vi "Histogram Main.vi"() -> ()   [LabVIEW 2022 SP3]
uses:
  Consumer Message.ctl
  <vilib>/Utility/file.llb/Write Delimited Spreadsheet (DBL).vi
  <vilib>/ErrorRing/Error Ring.xnode
panel:
  out "Histogram":cluster{"histogram":dbl[], "x axis":dbl[]}(graph)
  in  "bins":i32=20
  in  "signal":u16(ring) items=["uniform white", "uniform+uniform", "Gaussian white", "sine", "square"]
  out "Consumer Shutdown?":bool
  out "Backlog":u8(slide) scale=0.0..100.0
  in  "Snapshot":bool
  in  "Stop":bool
  # "Number of enqueued messages waiting to be processed"
  # "Current data being processed in consumer loop"
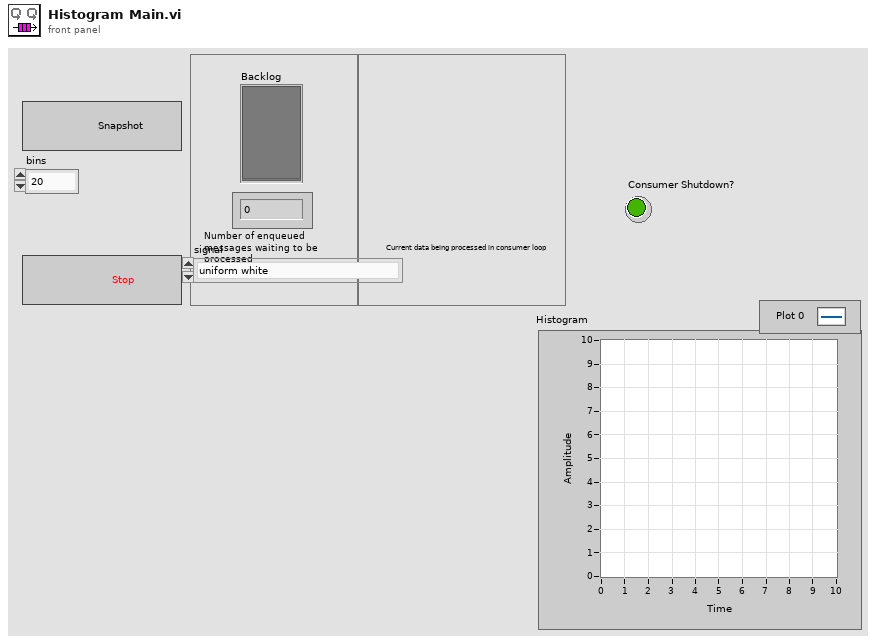
[diagram p1: front panel]
types:
  T1 = typedef "Consumer Message.ctl" = cluster{"Consumer State":string, "Boolean Data":bool, "Numeric Data":i32, "Signal":dbl[], "Error":errorcluster}
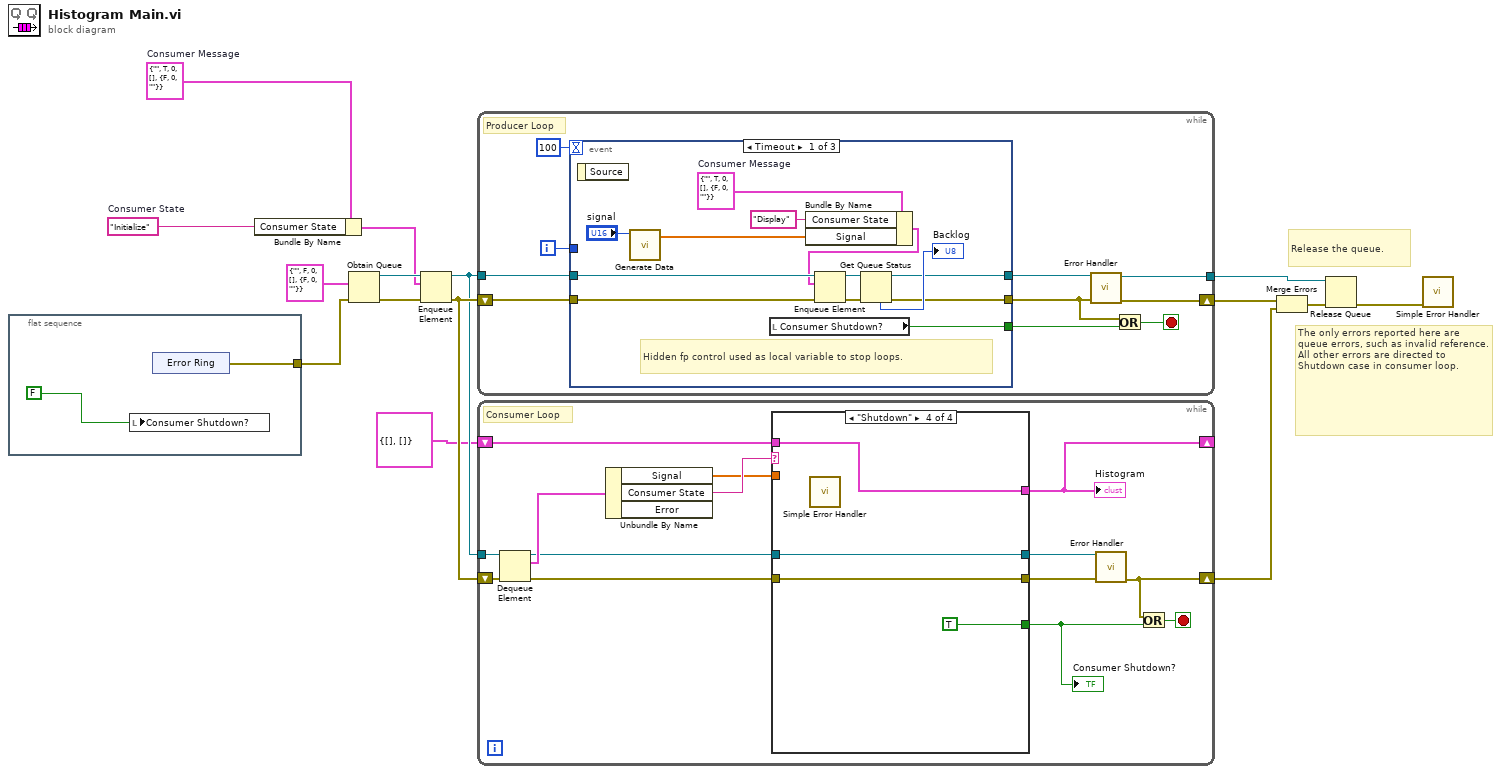
[diagram p0: block diagram]
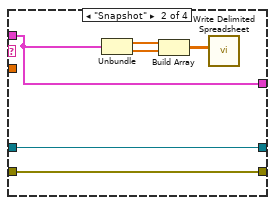
[diagram p3: hidden frame]
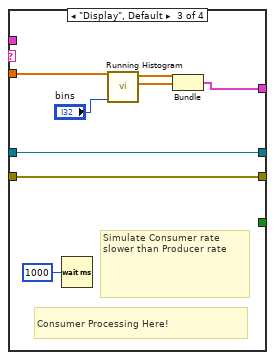
[diagram p4: hidden frame]
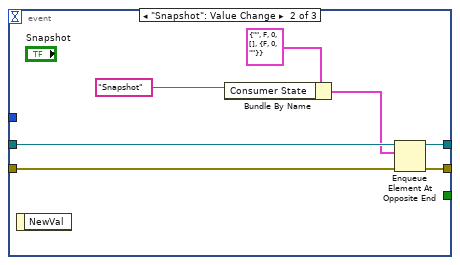
[diagram p5: hidden frame]
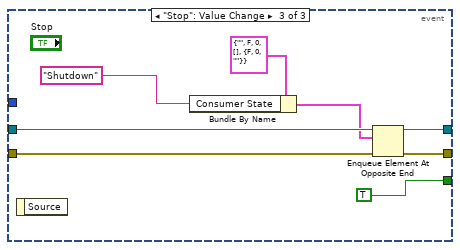
[diagram p6: hidden frame]
diagram:
  w7 = "Initialize"  # Consumer State
  w9 = T1 {"Consumer State"="", "Boolean Data"=TRUE, "Numeric Data"=0, "Signal"=[], "Error"={"status"=FALSE, "code"=0, "source"=""}}  # Consumer Message
  # "Release the queue."
  # "The only errors reported here are queue errors, such as invalid reference.  All other errors are directed to Shutdown case in consumer loop."
  n1 = flat-sequence {
    tunnel: [w16] -> w10
    frame #0 {
      n2 = local write "Consumer Shutdown?"(FALSE ("Stop Loops (local)")) -> ()
      n3 = xnode "Error Ring"() -> ("error out"=w16:errorcluster)
    }
  }
  n4 = Bundle By Name(cluster=w9, "Consumer State"=w7) -> (w8:T1)
  n5 = Obtain Queue(element data type=T1 {"Consumer State"="", "Boolean Data"=FALSE, "Numeric Data"=0, "Signal"=[], "Error"={"status"=FALSE, "code"=0, "source"=""}}, error in (no error)=w10) -> (queue out=w12:refnum<queue>, error out=w15:errorcluster)  [unwired: 3 in, 1 out]
  n6 = Enqueue Element(queue=w12, element=w8, error in (no error)=w15) -> (queue out=w11:refnum<queue>, error out=w13:errorcluster)  [unwired: 1 in, 1 out]
  n7 = while {
    tunnel: w11 -> [w28]
    shift-right: [w20] -> w6
    shift-left: w13 -> [w27]
    tunnel: [w19] -> w2
    i -> [w26]
    stop <- w22 stop-if-true
    # "Producer Loop"
    n8 = event shown="[0] Timeout" {
      selector: _ -> [_ _ _]
      dyn-events: _ -> [_ _ _]
      timeout: 100 -> [_ _ _]
      tunnel: w28 -> [w38 w46 w55]
      tunnel: w27 -> [w37 w45 w53]
      tunnel: [w36 w47 w52] -> w21
      tunnel: [w40 _ TRUE] -> w23
      tunnel: w26 -> [_ _ _]
      tunnel: [w35 w42 w51] -> w25
      event Timeout {
        w34 = T1 {"Consumer State"="", "Boolean Data"=TRUE, "Numeric Data"=0, "Signal"=[], "Error"={"status"=FALSE, "code"=0, "source"=""}}  # Consumer Message
        # "Hidden fp control used as local variable to stop loops."
        n9 = event-data() -> ()  [unwired: 1 in, 1 out]
        n10 = call "Generate Data.vi"("signal"="signal") -> ("Y"=w33:dbl[])  [unwired: 9 in, 1 out]
        n11 = local read "Consumer Shutdown?"() -> (w40:bool)
        n12 = Bundle By Name(cluster=w34, "Consumer State"="Display", "Signal"=w33) -> (w29:T1)
        n13 = Enqueue Element(queue=w38, element=w29) -> (queue out=w30:refnum<queue>)  [unwired: 2 in, 2 out]
        n14 = Get Queue Status(queue=w30, error in (no error)=w37) -> (queue out=w35:refnum<queue>, error out=w36:errorcluster, # elements in queue=→"Backlog":i32)  [unwired: 1 in, 5 out]
      }
      event "Snapshot": Value Change {
        n15 = event-data() -> ()  [unwired: 1 in, 1 out]
        n16 = Bundle By Name(cluster=T1 {"Consumer State"="", "Boolean Data"=FALSE, "Numeric Data"=0, "Signal"=[], "Error"={"status"=FALSE, "code"=0, "source"=""}}, "Consumer State"="Snapshot" ("String Data")) -> (w43:T1)
        n17 = Enqueue Element At Opposite End(queue=w46, element=w43, error in (no error)=w45) -> (queue out=w42:refnum<queue>, error out=w47:errorcluster)  [unwired: 1 in, 1 out]
      }
      event "Stop": Value Change {
        n18 = event-data() -> ()  [unwired: 1 in, 1 out]
        n19 = Bundle By Name(cluster=T1 {"Consumer State"="", "Boolean Data"=FALSE, "Numeric Data"=0, "Signal"=[], "Error"={"status"=FALSE, "code"=0, "source"=""}}, "Consumer State"="Shutdown") -> (w48:T1)
        n20 = Enqueue Element At Opposite End(queue=w55, element=w48, error in (no error)=w53) -> (queue out=w51:refnum<queue>, error out=w52:errorcluster)  [unwired: 1 in, 1 out]
      }
    }
    n21 = call "Error Handler.vi"("error in"=w21, "queue in"=w25) -> ("error out"=w20:errorcluster, "queue out"=w19:refnum<queue>)  [unwired: 8 in]
    n22 = Or(x=w21, y=w23) -> (x .or. y?=w22:bool)
  }
  n23 = while {
    tunnel: w11 -> [w69]
    shift-right: [w62] -> w5
    shift-left: w13 -> [w68]
    shift-right: [w57] -> _
    shift-left: cluster{"histogram":dbl[], "x axis":dbl[]} {"histogram"=[], "x axis"=[]} -> [w56]
    stop <- w63 stop-if-true
    # "Consumer Loop"
    n24 = Dequeue Element(queue=w69, error in (no error)=w68) -> (queue out=w61:refnum<queue>, element=w67:T1, error out=w60:errorcluster)  [unwired: 1 in, 1 out]
    n25 = Unbundle By Name(w67) -> ("Signal"=w58:dbl[], "Consumer State"=w59:string)  [unwired: 1 out]
    n26 = case shown="\"Shutdown\"" w59 {
      tunnel: [_ _ _ TRUE] -> w64
      tunnel: w60 -> [w71 w77 w84 w88]
      tunnel: [w71 w77 w84 w88] -> w66
      tunnel: w61 -> [w72 w78 w86 w89]
      tunnel: [w72 w78 w86 w89] -> w65
      tunnel: w58 -> [_ _ w83 _]
      tunnel: [w70 w76 w79 w87] -> w57
      tunnel: w56 -> [w70 w76 _ w87]
      frame "Initialize" {
      }
      frame "Snapshot" {
        n27 = Unbundle(w76) -> ("histogram"=w75:dbl[], "x axis"=w74:dbl[])
        n28 = Build Array(w75, w74) -> (w73:dbl[][])
        n29 = call-poly <vilib>:"Write Delimited Spreadsheet.vi"("2D data"=w73) -> ()  [unwired: 13 in, 2 out]
      }
      frame "Display", Default {
        # "Simulate Consumer rate slower than Producer rate"
        # "Consumer Processing Here!"
        n30 = Wait (ms)(milliseconds to wait=u32 1000) -> ()  [unwired: 1 out]
        n31 = call "Running Histogram.vi"("bins"="bins", "input data"=w83) -> ("x axis"=w80:dbl[], "histogram"=w81:dbl[])  [unwired: 6 in, 2 out]
        n32 = Bundle("histogram"=w81, "x axis"=w80) -> (w79:cluster{"histogram":dbl[], "x axis":dbl[]})  [unwired: 1 in]
      }
      frame "Shutdown" {
        n33 = call <vilib>:"Simple Error Handler.vi"() -> ()  [unwired: 5 in, 5 out]
      }
    }
    "Consumer Shutdown?" <- w64
    "Histogram" <- w57
    n34 = call "Error Handler.vi"("error in"=w66, "queue in"=w65) -> ("error out"=w62:errorcluster)  [unwired: 8 in, 1 out]
    n35 = Or(x=w62, y=w64) -> (x .or. y?=w63:bool)
  }
  n36 = Merge Errors(w6, w5) -> (w4:errorcluster)
  n37 = Release Queue(queue=w2, error in (no error)=w4) -> (error out=w3:errorcluster)  [unwired: 1 in, 2 out]
  n38 = call <vilib>:"Simple Error Handler.vi"("error in (no error)"=w3) -> ()  [unwired: 4 in, 5 out]
